vi "Set LibraryPaths to Include Icon Editor.vi"(8 "error in (no error)":errorcluster) -> (0 "error out":errorcluster, 3 "config modified?":bool)   [LabVIEW 2020]
uses:
  <vilib>/Utility/config.llb/Read Key (String).vi
  <vilib>/Utility/config.llb/Write Key (String).vi
  <vilib>/Utility/config.llb/NI_LVConfig.lvlib
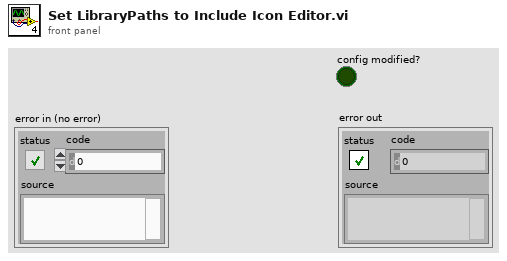
[diagram p1: front panel]
types:
  T1 = typedef "NI_LVConfig.lvlib/Config Data RefNum.ctl" = refnum<k1>
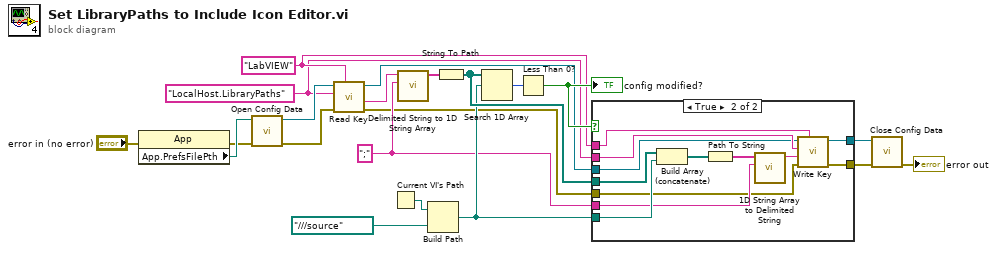
[diagram p0: block diagram]
diagram:
  w11 = ";" ("delimiter")
  w10 = "LabVIEW" ("section")
  w9 = "LocalHost.LibraryPaths" ("key")
  n1 = property class="App"(error in="error in (no error)") -> (error out=w6:errorcluster, "App.PrefsFilePth"=w21:path)  [unwired: 1 in, 1 out]
  n2 = call <vilib>:"Open Config Data.vi"("error in (no error)"=w6, "configuration file path"=w21) -> ("error out"=w7:errorcluster, "refnum"=w20:T1)  [unwired: 7 in, 1 out]
  n3 = call-poly <vilib>:"Read Key.vi"("section"=w10, "error in (no error)"=w7, "key"=w9, "refnum"=w20) -> ("error out"=w5:errorcluster, "value"=w17:string, "refnum out"=w8:T1)  [unwired: 4 in, 1 out]
  n4 = Current VI's Path() -> (path=w18:path)
  n5 = call <vilib>:"Delimited String to 1D String Array.vi"("delimiter"=w11, "delimited string"=w17) -> ("string array"=w16:string[])  [unwired: 9 in]
  n6 = Build Path(base path=w18, name or relative path=path "../../../source") -> (appended path=w12:path)
  n7 = String To Path(string=w16) -> (path=w13:path[])
  n8 = Search 1D Array(1D array=w13, element=w12) -> (index of element=w15:i32)  [unwired: 1 in]
  n9 = Less Than 0?(x=w15) -> (x < 0?=w14:bool)
  "config modified?" <- w14
  n10 = case shown="True" w14 {
    tunnel: w13 -> [_ w35]
    tunnel: w12 -> [_ w34]
    tunnel: w11 -> [_ w31]
    tunnel: w10 -> [_ w30]
    tunnel: w9 -> [_ w29]
    tunnel: w8 -> [w23 w27]
    tunnel: w5 -> [w22 w26]
    tunnel: [w23 w25] -> w4
    tunnel: [w22 w24] -> w3
    frame False {
    }
    frame True {
      n11 = Build Array (concatenate)(w35, w34) -> (w33:path[])
      n12 = Path To String(path=w33) -> (string=w32:string[])
      n13 = call <vilib>:"1D String Array to Delimited String.vi"("delimiter"=w31, "string array"=w32) -> ("delimited string"=w28:string)  [unwired: 9 in]
      n14 = call-poly <vilib>:"Write Key.vi"("section"=w30, "error in (no error)"=w26, "value"=w28, "key"=w29, "refnum"=w27) -> ("error out"=w24:errorcluster, "refnum out"=w25:T1)  [unwired: 4 in, 1 out]
    }
  }
  n15 = call <vilib>:"Close Config Data.vi"("error in (no error)"=w3, "refnum"=w4) -> ("error out"=→"error out":errorcluster)  [unwired: 8 in, 1 out]
